vi "截取CRC.vi"(5 "字符串":string) -> (1 "CRC":string)   [LabVIEW 2016, in "数据传输系统-04.lvlib" / "自动更新.lvlib" / "TCP文件传输系统.lvlib" / "TCP接收文件.lvlib"]
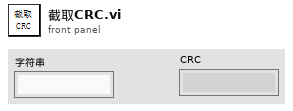
[diagram p1: front panel]
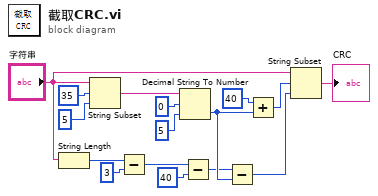
[diagram p0: block diagram]
diagram:
  n1 = String Length(string="字符串") -> (length=w15:i32)
  n2 = String Subset(string="字符串", offset (0)=35 ("偏移量(0)"), length (rest)=5 ("长度（剩余）")) -> (substring=w8:string)
  n3 = Subtract(x=w15, y=3) -> (x-y=w5:i32)
  n4 = Decimal String To Number(string=w8, offset=0 ("偏移量"), default (0L)=5 ("默认(0 I32)")) -> (number=w14:i32)  [unwired: 1 out]
  n5 = Subtract(x=w5, y=40) -> (x-y=w11:i32)
  n6 = Subtract(x=w11, y=w14) -> (x-y=w3:i32)
  n7 = Add(x=40 ("偏移量(0)"), y=w14) -> (x+y=w4:i32)
  n8 = String Subset(string="字符串", offset (0)=w4, length (rest)=w3) -> (substring=→"CRC":string)
